vi "2-3.vi"() -> ()   [LabVIEW 2018]
uses:
  <vilib>/Analysis/3filter.llb/Filter Passband Type.ctl
  <vilib>/Analysis/3filter.llb/Butterworth Filter (DBL).vi
  <vilib>/express/express analysis/Spectral/Block/exnSpectralBlock spectral measurements peak poly.vi
  <vilib>/express/express analysis/Spectral/Block/exnSpectralBlock spectral measurements peak WFM.vi
  <vilib>/express/express analysis/Spectral/XNode/ExpressSpectralMeasurementsBlockNode.xnode
  <vilib>/measure/NI_MABase.lvlib
  <vilib>/Analysis/NI_AALPro.lvlib
  <vilib>/Analysis/NI_AALBase.lvlib
panel:
  in  "停止":bool
  in  "带通Butterworth滤波器":cluster{"中心频率(Hz)":dbl, "带宽(Hz)":dbl}={"中心频率(Hz)"=150000.0, "带宽(Hz)"=280000.0}
  out "fh":dbl
  out "fl":dbl
  in  "选项卡控件":enum32{"调制", "滤波", "解调"}(tab)
  out "频域":cluster{"f0":dbl, "df":dbl, "magnitude":dbl[]}(graph)
  out "时域":waveform(dbl)[](graph)
  out "频域":cluster{"f0":dbl, "df":dbl, "magnitude":dbl[]}(graph)
  out "时域":waveform(dbl)(graph)
  out "时域 2":waveform(dbl)[](graph)
  out "BT(Hz)":dbl
  out "数组":dbl[](array[numeric])
  out "调制信号":waveform(dbl)(graph)
  out "积分信号":waveform(dbl)(graph)
  out "采样参数（采样频率fs，采样数Ns）":cluster{dbl, dbl} {"?" format="%#_6f"; "?" format="%#_6f"}
  out "载波信号":waveform(dbl)(graph)
  in  "kf(Hz/V)":dbl=50000.0
  in  "An(V)":dbl=0.1
  in  "调制信号":cluster{"T(s)":dbl, "Am(V)":dbl}={"T(s)"=0.0002, "Am(V)"=1.0}
  in  "载波信号":cluster{"fc(Hz)":dbl, "Ac(V)":dbl}={"fc(Hz)"=150000.0, "Ac(V)"=1.0}
  # "要显示n个周期的调制信号波形，\n则采样数Ns=n*fs/fm"
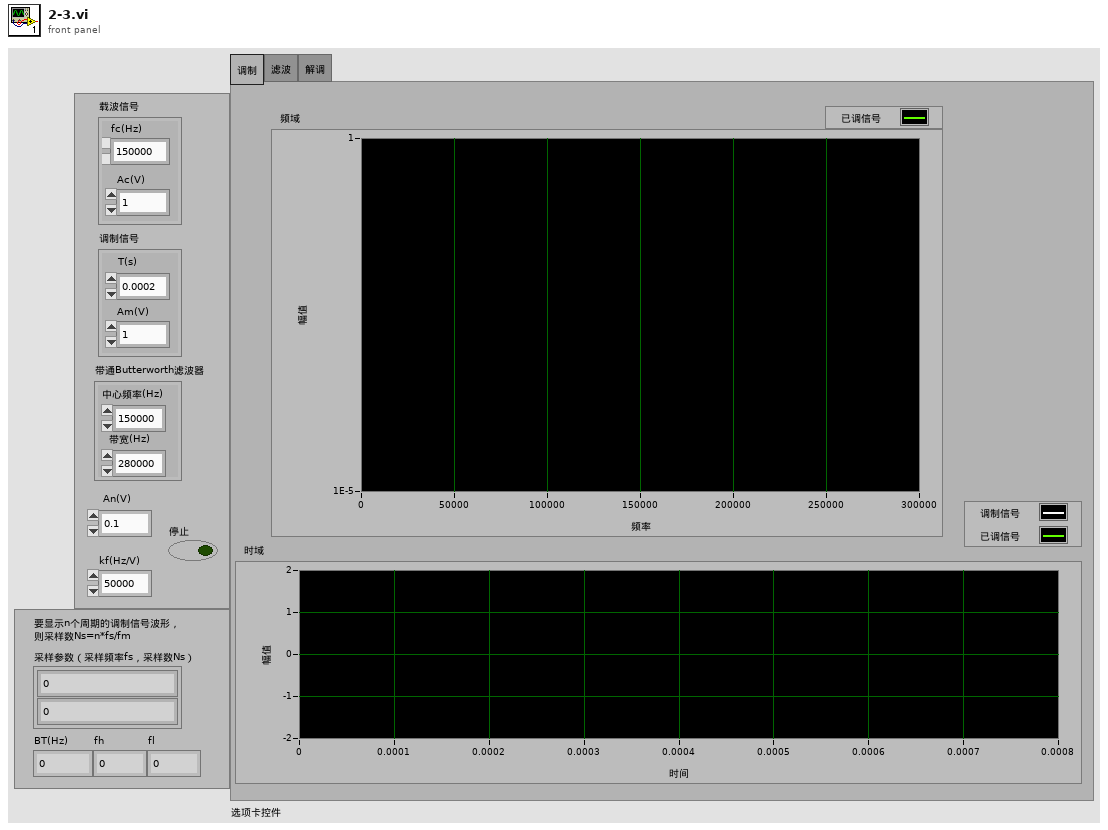
[diagram p1: front panel]
types:
  T1 = typedef "NI_AALBase.lvlib/Filter Passband Type.ctl" = enum32{"Lowpass", "Highpass", "Bandpass", "Bandstop"}
  T2 = cluster{"averaging mode":u16, "weighting mode":u16, "number of averages":u32}
  T3 = cluster{"dB On (F)":bool, "unwrap phase (F)":bool, "convert to degree (F)":bool}
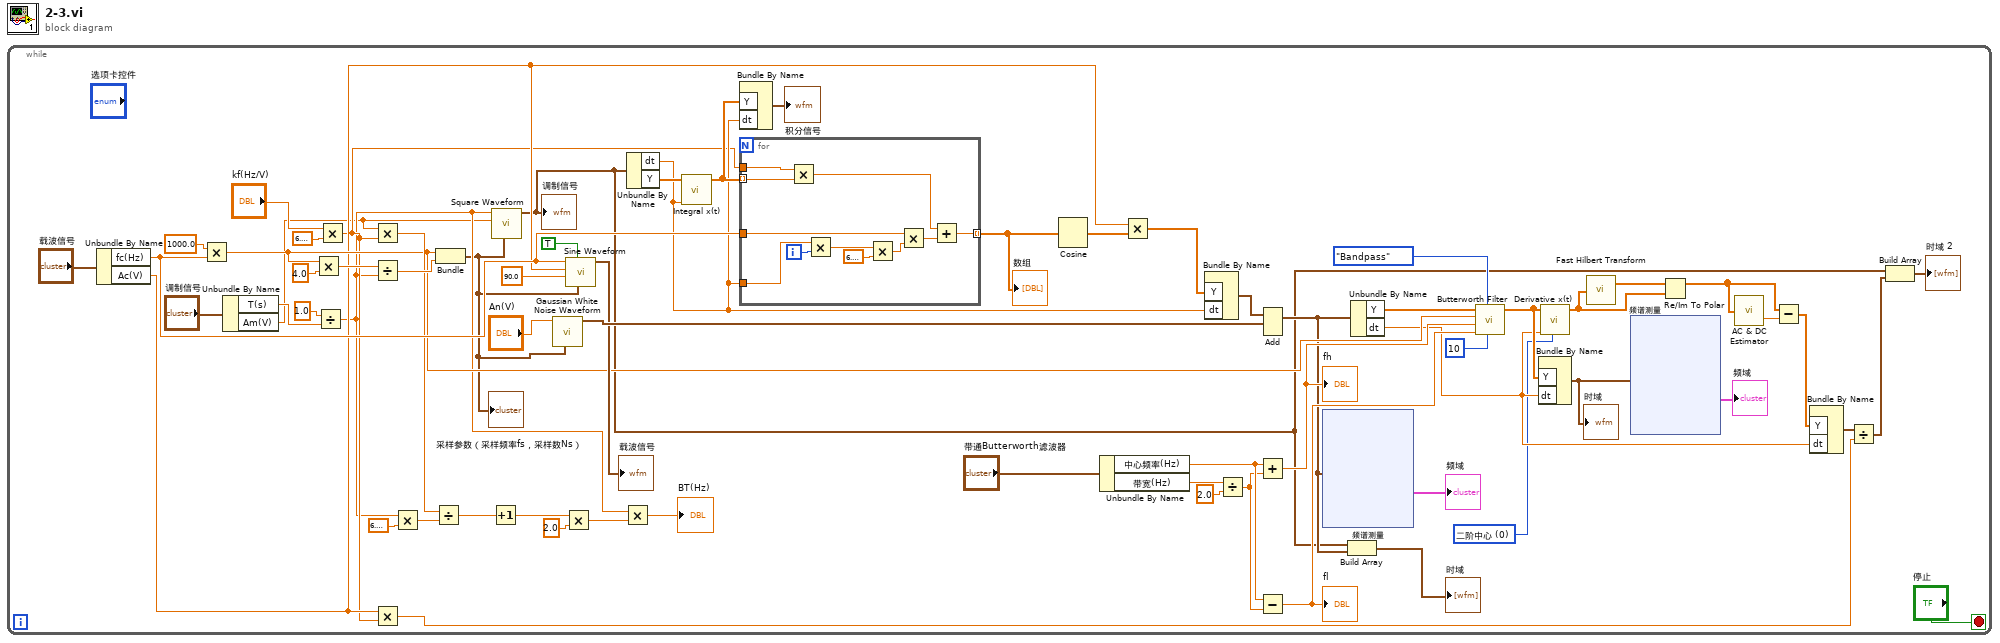
[diagram p0: block diagram]
diagram:
  n1 = while {
    stop <- "停止" stop-if-true
    w19 = u16 0 items=["二阶中心", "四阶中心", "前向", "后向"] ("method")
    n2 = Unbundle By Name("载波信号") -> ("fc(Hz)"=w55:dbl, "Ac(V)"=w15:dbl)
    n3 = Multiply(x=1000.0, y=w55) -> (x*y=w27:dbl)
    n4 = Unbundle By Name("调制信号") -> ("T(s)"=w5:dbl, "Am(V)"=w3:dbl)
    n5 = Multiply(x=w27, y=4.0) -> (x*y=w61:dbl)
    n6 = Divide(x=1.0, y=w5) -> (x/y=w4:dbl)
    n7 = Multiply(x="kf(Hz/V)", y=6.283185307179586) -> (x*y=w9:dbl)
    n8 = Multiply(x=w3, y=w9) -> (x*y=w42:dbl)
    n9 = Divide(x=w61, y=w4) -> (x/y=w60:dbl)
    n10 = Multiply(x=w15, y=w9) -> (x*y=w13:dbl)
    n11 = Multiply(x=w4, y=6.283185307179586) -> (x*y=w43:dbl)
    n12 = Divide(x=w42, y=w43) -> (x/y=w41:dbl)
    n13 = Bundle(w27, w60) -> (w2:cluster{dbl, dbl})  [unwired: 1 in]
    "采样参数（采样频率fs，采样数Ns）" <- w2
    n14 = Increment(x=w41) -> (x+1=w40:dbl)
    n15 = call <vilib>:"Square Waveform.vi"("sampling info"=w2, "amplitude"=w3, "frequency"=w4) -> ("signal out"=w1:waveform(dbl))  [unwired: 7 in, 1 out]
    "调制信号" <- w1
    n16 = call <vilib>:"Gaussian White Noise Waveform.vi"("sampling info"=w2, "standard deviation"="An(V)") -> ("signal out"=w47:waveform(dbl))  [unwired: 8 in, 1 out]
    n17 = Multiply(x=w40, y=2.0) -> (x*y=w38:dbl)
    n18 = call <vilib>:"Sine Waveform.vi"("sampling info"=w2, "reset signal"=TRUE, "phase"=90.0, "amplitude"=w15, "frequency"=w55) -> ("signal out"=→"载波信号":waveform(dbl))  [unwired: 5 in, 1 out]
    n19 = Multiply(x=w4, y=w38) -> (x*y=→"BT(Hz)":dbl)
    n20 = Unbundle By Name(w1) -> ("dt"=w52:dbl, "Y"=w62:dbl[])
    n21 = call <vilib>:"Integral x(t).vi"("dt"=w52, "X"=w62) -> ("Integral X"=w56:dbl[])  [unwired: 8 in, 1 out]
    n22 = Bundle By Name("Y"=w56, "dt"=w52) -> (→"积分信号":waveform(dbl))  [unwired: 1 in]
    n23 = for {
      tunnel: w56 -> [w98] mode=indexing
      tunnel: w52 -> [w96]
      tunnel: w55 -> [w92]
      tunnel: [w89] -> w54 mode=indexing
      tunnel: w9 -> [w88]
      i -> [w97]
      n24 = Multiply(x=w88, y=w98) -> (x*y=w90:dbl)
      n25 = Multiply(x=w96, y=w97) -> (x*y=w94:dbl)
      n26 = Multiply(x=w94, y=6.283185307179586) -> (x*y=w93:dbl)
      n27 = Multiply(x=w92, y=w93) -> (x*y=w91:dbl)
      n28 = Add(x=w90, y=w91) -> (x+y=w89:dbl)
    }
    "数组" <- w54
    n29 = Cosine(x=w54) -> (cos(x)=w53:dbl[])
    n30 = Unbundle By Name("带通Butterworth滤波器") -> ("中心频率(Hz)"=w29:dbl, "带宽(Hz)"=w33:dbl)
    n31 = Multiply(x=w15, y=w53) -> (x*y=w51:dbl[])
    n32 = Bundle By Name("Y"=w51, "dt"=w52) -> (w49:waveform(dbl))  [unwired: 1 in]
    n33 = Divide(x=w33, y=2.0) -> (x/y=w28:dbl)
    n34 = Add(1:w47, 2:w49) -> (0:w25:waveform(dbl))  [unwired: 1 in, 1 out]
    n35 = Add(x=w29, y=w28) -> (x+y=w31:dbl)
    "fh" <- w31
    n36 = Subtract(x=w29, y=w28) -> (x-y=w30:dbl)
    "fl" <- w30
    n37 = xnode "频谱测量"("信号"=w25) -> ("FFT - （峰值）"=→"频域":cluster{"f0":dbl, "df":dbl, "magnitude":dbl[]})  [unwired: 1 in, 2 out]
    n38 = Build Array(w1, w25) -> (→"时域":waveform(dbl)[])
    n39 = Unbundle By Name(w25) -> ("Y"=w24:dbl[], "dt"=w20:dbl)
    n40 = call-poly <vilib>:"Butterworth Filter.vi"("order"=10, "filter type"=Filter_Passband_Type."Bandpass", "low cutoff freq: fl"=w30, "high cutoff freq: fh"=w31, "sampling freq: fs"=w27, "X"=w24) -> ("Filtered X"=w22:dbl[])  [unwired: 2 in, 1 out]
    n41 = Bundle By Name("Y"=w22, "dt"=w20) -> (w23:waveform(dbl))  [unwired: 1 in]
    "时域" <- w23
    n42 = call <vilib>:"Derivative x(t).vi"("method"=w19, "dt"=w20, "X"=w22) -> ("dX/dt"=w12:dbl[])  [unwired: 7 in, 1 out]
    n43 = call <vilib>:"Fast Hilbert Transform.vi"("X"=w12) -> ("Hilbert{X}"=w21:dbl[])  [unwired: 1 out]
    n44 = xnode "频谱测量"("信号"=w23) -> ("FFT - （峰值）"=→"频域":cluster{"f0":dbl, "df":dbl, "magnitude":dbl[]})  [unwired: 1 in, 2 out]
    n45 = Re/Im To Polar(2:w12, 3:w21) -> (1:w18:dbl[])  [unwired: 1 out]
    n46 = call <vilib>:"AC & DC Estimator.vi"("Signal (V)"=w18) -> ("DC estimate (V)"=w17:dbl)  [unwired: 1 out]
    n47 = Subtract(x=w18, y=w17) -> (x-y=w16:dbl[])
    n48 = Bundle By Name("Y"=w16, "dt"=w20) -> (w14:waveform(dbl))  [unwired: 1 in]
    n49 = Divide(x=w14, y=w13) -> (x/y=w8:waveform(dbl))
    n50 = Build Array(w1, w8) -> (→"时域 2":waveform(dbl)[])
  }
